vi "Create Test Library from Template.vi"() -> ()   [LabVIEW 2016]
doc: "This VI creates and adds the Drona test library template to the active project"
uses:
  _SubVIs/ScriptSubVIs.lvlib
panel:
  out "error out":errorcluster
  in  "error in (no error)":errorcluster
  in  "VIs to include":string[](array[string])=["Run.vi", "TestTemplate.vi"]
  in  "Library Name":string="TestLibraryTemplate.lvlib"
  # "Creating Drona Test Library\nfrom Template......"
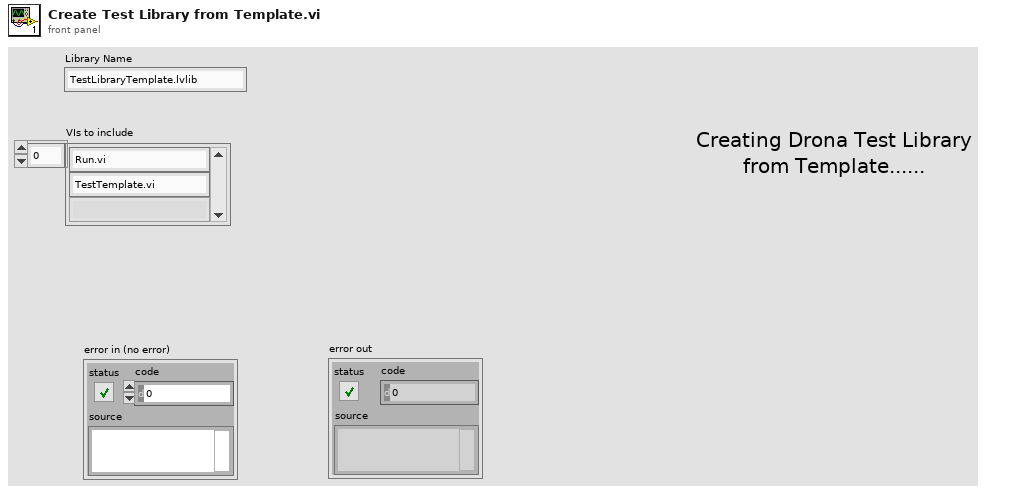
[diagram p1: front panel]
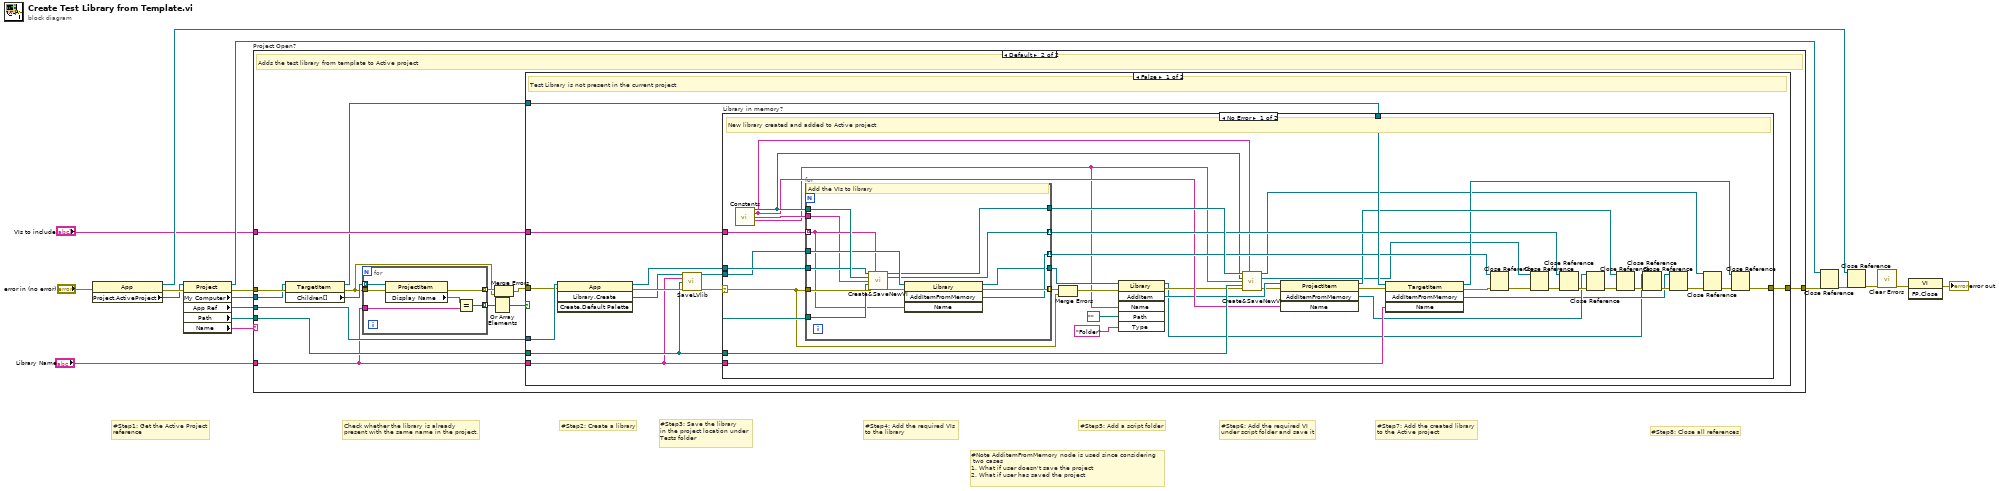
[diagram p0: block diagram]
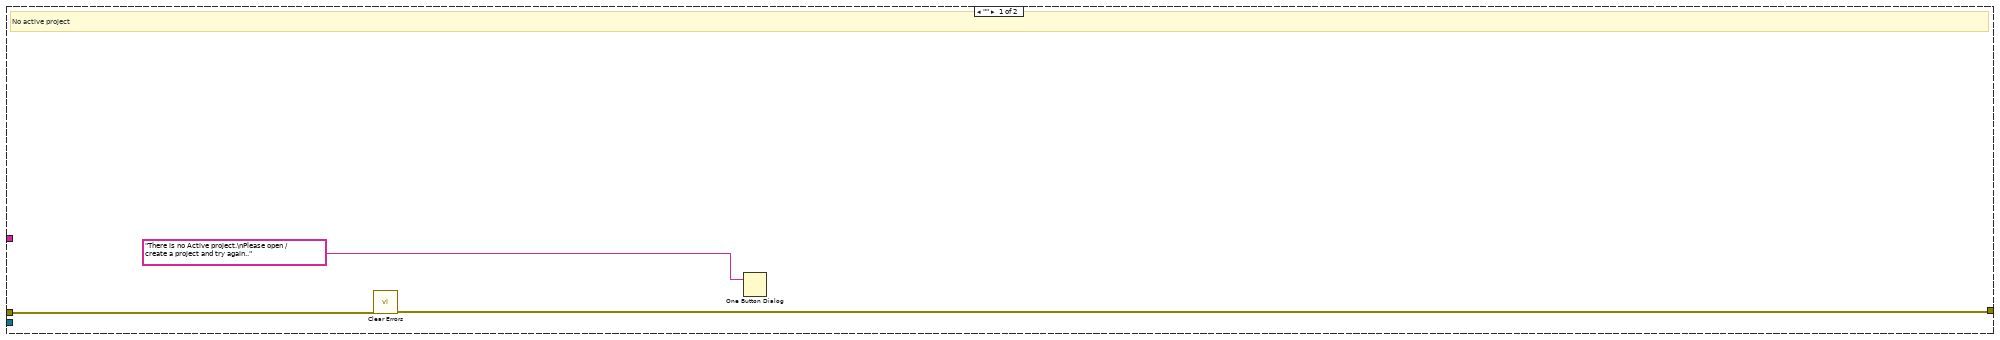
[diagram p2: hidden frame]
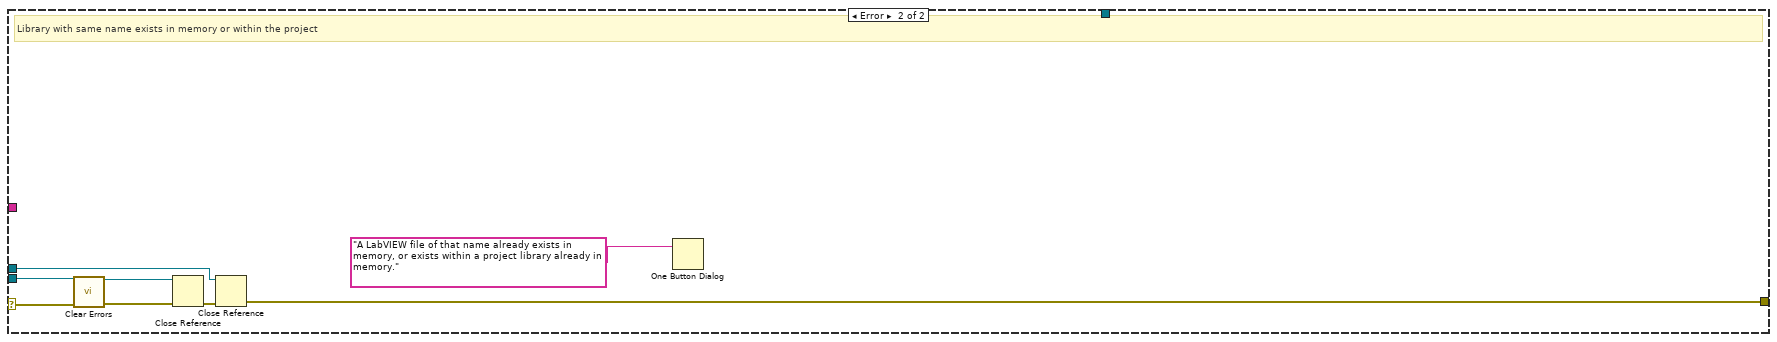
[diagram p3: hidden frame]
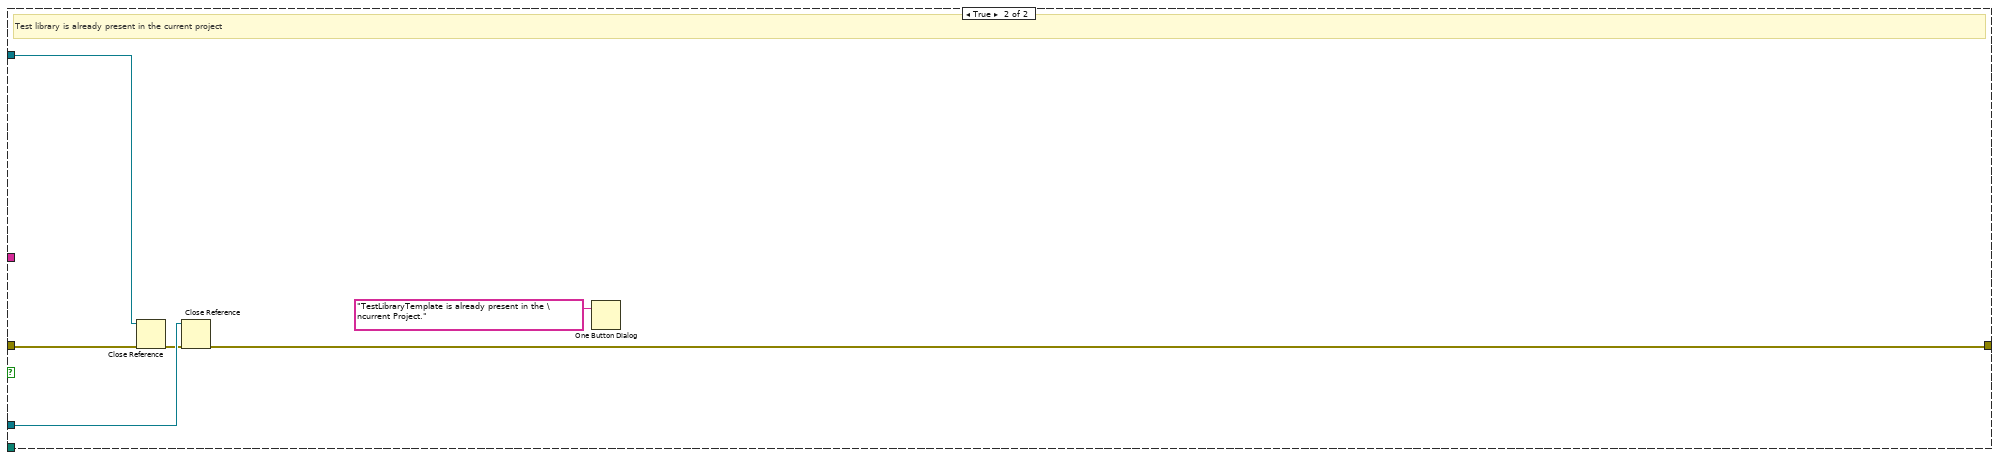
[diagram p4: hidden frame]
diagram:
  # "Check whether the library is already \npresent with the same name in the project."
  # "#Note AdditemFromMemory node is used since considering\n two cases  \n1. What if user doesn't save the project\n2. What if user has saved the project"
  # "#Step8: Close all references"
  # "#Step7: Add the created library\nto the Active project"
  # "#Step6: Add the required VI \nunder script folder and save it"
  # "#Step5: Add a script folder"
  # "#Step4: Add the required VIs \nto the library"
  # "#Step3: Save the library \nin the project location under \nTests folder"
  # "#Step2: Create a library"
  # "#Step1: Get the Active Project\nreference"
  n1 = property class="App"(error in="error in (no error)") -> (reference out=w12:refnum<vi>, error out=w17:errorcluster, "Project.ActiveProject"=w11:refnum<vi>)  [unwired: 1 in]
  n2 = property class="Project"(reference=w11, error in=w17) -> (reference out=w10:refnum<vi>, error out=w16:errorcluster, "My Computer"=w1:refnum<vi>, "App Ref"=w15:refnum<vi>, "Path"=w9:path, "Name"=w8:string)
  n3 = case "Project Open?" shown="Default" w8 {
    tunnel: w1 -> [_ w29]
    tunnel: w16 -> [w20 w30]
    tunnel: w15 -> [_ w33]
    tunnel: [w19 w31] -> w14
    tunnel: w9 -> [_ w34]
    tunnel: "Library Name" -> [_ w26]
    tunnel: "VIs to include" -> [_ w32]
    frame "" {
      # "No active project"
      n4 = call <vilib>:"Clear Errors.vi"("error in (no error)"=w20) -> ("error out"=w19:errorcluster)  [unwired: 5 in, 1 out]
      n5 = One Button Dialog(message="There is no Active project.\nPlease open / create a project and try again..") -> ()  [unwired: 1 in, 1 out]
    }
    frame Default {
      # "Adds the test library from template to Active project"
      n6 = property class="TargetItem"(reference=w29, error in=w30) -> (reference out=w28:refnum<vi>, error out=w22:errorcluster, "Children[]"=w27:refnum<vi>[])
      n7 = for {
        tunnel: w27 -> [w118] mode=indexing
        tunnel: [w116] -> w25 mode=indexing
        tunnel: w26 -> [w115]
        tunnel: w22 -> [w114]
        tunnel: [w113] -> w23 mode=indexing
        n8 = property class="ProjectItem"(reference=w118, error in=w114) -> (error out=w113:errorcluster, "Display Name"=w117:string)  [unwired: 1 out]
        n9 = Equal?(x=w117, y=w115) -> (x = y?=w116:bool)
      }
      n10 = Or Array Elements(Boolean array=w25) -> (logical OR=w24:bool)
      n11 = Merge Errors(w23, w22) -> (w21:errorcluster)
      n12 = case shown="False" w24 {
        tunnel: w34 -> [w44 _]
        tunnel: w33 -> [w43 w110]
        tunnel: w32 -> [w42 _]
        tunnel: [w39 w108] -> w31
        tunnel: w28 -> [w37 w111]
        tunnel: w26 -> [w36 _]
        tunnel: w21 -> [w35 w112]
        frame False {
          # "Test Library is not present in the current project"
          n13 = invoke class="App" method="Library.Create"(reference=w43, error in=w35) -> (reference out=w40:refnum<vi>, error out=w46:errorcluster, "Create Library"=w45:refnum<vi>)  [unwired: 2 in, 1 out]
          n14 = call "SaveLVlib.vi"("Library in"=w45, "Library Name"=w36, "Project Path"=w44, "error in (no error)"=w46) -> ("Library out"=w38:refnum<vi>, "error out"=w41:errorcluster)  [unwired: 10 in]
          n15 = case "Library in memory?" shown="No Error" w41 {
            selector: w41 -> [w82 w106]
            tunnel: w44 -> [w86 _]
            tunnel: w37 -> [w85 _]
            tunnel: w36 -> [w84 _]
            tunnel: w42 -> [w83 _]
            tunnel: w40 -> [w81 w104]
            tunnel: [w80 w102] -> w39
            tunnel: w38 -> [w74 w105]
            frame No Error {
              # "New library created and added to Active project"
              n16 = call "Constants.vi"() -> ("VI path"=w72:path, "Exe script name"=w71:string, "Test folder name"=w70:string, "Script folder name"=w69:string)  [unwired: 12 in]
              n17 = for {
                tunnel: w72 -> [w98]
                tunnel: w83 -> [w93] mode=indexing
                tunnel: w82 -> [w99]
                tunnel: w81 -> [w97]
                tunnel: w74 -> [w96]
                tunnel: [w95] -> w79 mode=indexing
                tunnel: w86 -> [w94]
                tunnel: [w91] -> w76 mode=indexing
                tunnel: w70 -> [w90]
                tunnel: [w89] -> w77
                tunnel: [w88] -> w75 mode=indexing
                tunnel: [w87] -> w73
                # "Add the VIs to library"
                n18 = call "Create&SaveNewVI.vi"("Application ref in"=w97, "VI name"=w93, "VI path"=w98, "Folder name"=w90, "Project Path"=w94, "error in (no error)"=w99) -> ("Application ref out"=w89:refnum<vi>, "VI ref out"=w91:refnum<vi>, "error out"=w92:errorcluster)  [unwired: 7 in]
                n19 = invoke class="Library" method="AddItemFromMemory"(reference=w96, error in=w92, "Name"=w93) -> (reference out=w87:refnum<vi>, error out=w95:errorcluster, "AddItemFromMemory"=w88:refnum<vi>)  [unwired: 1 in, 1 out]
              }
              n20 = Merge Errors(w79, w82) -> (w78:errorcluster)
              n21 = invoke class="Library" method="AddItem"(reference=w73, error in=w78, "Name"=w69, "Path"=path "", "Type"="Folder") -> (reference out=w50:refnum<vi>, error out=w64:errorcluster, "AddItem"=w65:refnum<vi>)  [unwired: 1 in, 3 out]
              n22 = call "Create&SaveNewVI.vi"("Application ref in"=w77, "VI name"=w71, "VI path"=w72, "Folder name"=w69, "Project Path"=w86, "error in (no error)"=w64) -> ("Application ref out"=w49:refnum<vi>, "VI ref out"=w54:refnum<vi>, "error out"=w63:errorcluster)  [unwired: 7 in]
              n23 = invoke class="ProjectItem" method="AddItemFromMemory"(reference=w65, error in=w63, "Name"=w71) -> (reference out=w59:refnum<vi>, error out=w66:errorcluster, "AddItemFromMemory"=w60:refnum<vi>)  [unwired: 1 in, 1 out]
              n24 = invoke class="TargetItem" method="AddItemFromMemory"(reference=w85, error in=w66, "Name"=w84) -> (reference out=w55:refnum<vi>, error out=w48:errorcluster, "AddItemFromMemory"=w56:refnum<vi>)  [unwired: 1 in, 1 out]
              n25 = Close Reference(reference=w75, error in (no error)=w48) -> (error out=w47:errorcluster)
              n26 = Close Reference(reference=w54, error in (no error)=w47) -> (error out=w51:errorcluster)
              n27 = Close Reference(reference=w76, error in (no error)=w51) -> (error out=w62:errorcluster)
              n28 = Close Reference(reference=w60, error in (no error)=w62) -> (error out=w61:errorcluster)
              n29 = Close Reference(reference=w59, error in (no error)=w61) -> (error out=w58:errorcluster)
              n30 = Close Reference(reference=w50, error in (no error)=w58) -> (error out=w57:errorcluster)
              n31 = Close Reference(reference=w56, error in (no error)=w57) -> (error out=w53:errorcluster)
              n32 = Close Reference(reference=w49, error in (no error)=w53) -> (error out=w52:errorcluster)
              n33 = Close Reference(reference=w55, error in (no error)=w52) -> (error out=w80:errorcluster)
            }
            frame Error {
              # "Library with same name exists in memory or within the project"
              n34 = call <vilib>:"Clear Errors.vi"("error in (no error)"=w106) -> ("error out"=w103:errorcluster)  [unwired: 5 in, 1 out]
              n35 = Close Reference(reference=w105, error in (no error)=w103) -> (error out=w101:errorcluster)
              n36 = Close Reference(reference=w104, error in (no error)=w101) -> (error out=w102:errorcluster)
              n37 = One Button Dialog(message="A LabVIEW file of that name already exists in memory, or exists within a project library already in memory.") -> ()  [unwired: 1 in, 1 out]
            }
          }
        }
        frame True {
          # "Test library is already present in the current project"
          n38 = Close Reference(reference=w111, error in (no error)=w112) -> (error out=w109:errorcluster)
          n39 = Close Reference(reference=w110, error in (no error)=w109) -> (error out=w108:errorcluster)
          n40 = One Button Dialog(message="TestLibraryTemplate is already present in the \ncurrent Project.") -> ()  [unwired: 1 in, 1 out]
        }
      }
    }
  }
  n41 = Close Reference(reference=w10, error in (no error)=w14) -> (error out=w13:errorcluster)
  n42 = Close Reference(reference=w12, error in (no error)=w13) -> (error out=w5:errorcluster)
  n43 = call <vilib>:"Clear Errors.vi"("error in (no error)"=w5) -> ("error out"=w4:errorcluster)  [unwired: 5 in, 1 out]
  n44 = invoke class="VI" method="FP.Close"(error in=w4) -> (error out=→"error out":errorcluster)  [unwired: 2 in, 2 out]
